vi "Initialize From File.vi"(0 "NI Build Specification_LV in":refnum<class "NI Build Specification_LV.lvclass">) -> (4 "NI Build Specification_LV out":refnum<class "NI Build Specification_LV.lvclass">)   [LabVIEW 2017, in "CL_G3_VIComponentBuilder.lvlib" / "NI Build Specification_LV.lvclass"]
doc: "Initializes the class from the configuration file.\n <MustCallParent>Parent information must be read from file therefore overrides of this method must call the parent.</MustCallParent>"
uses:
  NI Build Specification_LV.lvclass
  C:/builds/Component BuilderBT/SrcDist/Exports/Exports/Export.lvclass
  Exports/Export.lvclass/Export.ctl
  NI Build Specification_LV.lvclass/NI Build Specification_LV.ctl
  Exports/Accessors/Read Export Operation Errors.vi
  Accessors/Read Export's Build Spec Name.vi
  Exports/Accessors/Read Export Config File.vi
  Exports/Accessors/Read Component Root path.vi
  Accessors/Write Build Number XML Prop Name.vi
  Accessors/Write Display Name XML Prop Name.vi
  Accessors/Write Unique Name XML Prop Name.vi
  Accessors/Write Build Spec Type.vi
  Accessors/Write Export's Build Spec Name.vi
  Accessors/Write Target Name Containing Build Specs to Build.vi
  Exports/Accessors/Write Export Operation Errors.vi
  Accessors/Write LabVIEW Project SubBuild Spec Order.vi
  <vilib>/Utility/error.llb/Error Cluster From Error Code.vi
  Exports/Export.lvclass
  <vilib>/Utility/config.llb/NI_LVConfig.lvlib
  CL_G3_VIComponentBuilder.lvlib
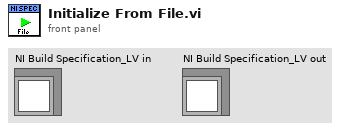
[diagram p1: front panel]
types:
  T1 = cluster{"Target Name Containing Build Specs to Build":string, "Sub Build Spec Order":path[], "Export's Build Spec Name":string}
  T2 = typedef "NI_LVConfig.lvlib/Config Data RefNum.ctl" = refnum<k1>
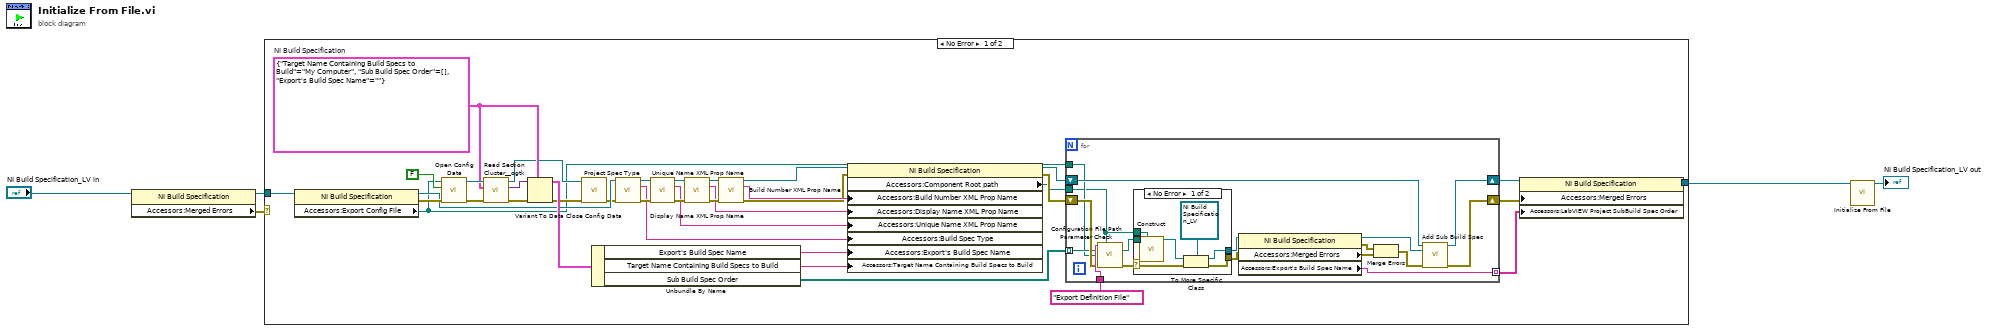
[diagram p0: block diagram]
diagram:
  n1 = property class="NI Build Specification"(reference="NI Build Specification_LV in") -> (reference out=w2:refnum<class "NI Build Specification_LV.lvclass">, "Accessors:Merged Errors"=w3:errorcluster)  [unwired: 1 in, 1 out]
  n2 = case shown="No Error" w3 {
    tunnel: [w12 w68] -> w1
    tunnel: w2 -> [w42 w68]
    frame No Error {
      w38 = T1 {"Target Name Containing Build Specs to Build"="My Computer", "Sub Build Spec Order"=[], "Export's Build Spec Name"=""}  # NI Build Specification
      n3 = property class="NI Build Specification"(reference=w42) -> (reference out=w30:refnum<class "NI Build Specification_LV.lvclass">, error out=w34:errorcluster, "Accessors:Export Config File"=w9:path)  [unwired: 1 in]
      n4 = call <vilib>:"Open Config Data.vi"("error in (no error)"=w34, "create file if necessary (T)"=FALSE, "configuration file path"=w9) -> ("error out"=w36:errorcluster, "refnum"=w40:T2)  [unwired: 6 in, 1 out]
      n5 = call <userlib>:"Read Section Cluster__ogtk.vi"("error in (no error)"=w36, "Section Formatted Cluster Type"=w38, "refnum"=w40) -> ("error out"=w35:errorcluster, "Section Formatted Cluster"=w39:variant, "dup refnum"=w33:T2)  [unwired: 4 in, 2 out]
      n6 = Variant To Data(error in=w35, type=w38, Variant=w39) -> (data=w37:T1, error out=w32:errorcluster)
      n7 = call <vilib>:"Close Config Data.vi"("error in (no error)"=w32, "refnum"=w33) -> ("error out"=w29:errorcluster)  [unwired: 8 in, 1 out]
      n8 = Unbundle By Name(w37) -> ("Export's Build Spec Name"=w8:string, "Target Name Containing Build Specs to Build"=w31:string, "Sub Build Spec Order"=w10:path[])
      n9 = call-dynamic "Project Spec Type.vi"("NI Build Specification in"=w30, "error in (no error)"=w29) -> ("NI Build Specification out"=w24:refnum<class "NI Build Specification_LV.lvclass">, "Project Specfication Type"=w17:string, "error out"=w21:errorcluster)  [unwired: 11 in]
      n10 = call-dynamic "Unique Name XML Prop Name.vi"("NI Build Specification in"=w24, "error in (no error)"=w21) -> ("NI Build Specification out"=w28:refnum<class "NI Build Specification_LV.lvclass">, "Unique Name XML Property Name"=w18:string, "error out"=w27:errorcluster)  [unwired: 11 in]
      n11 = call-dynamic "Display Name XML Prop Name.vi"("NI Build Specification in"=w28, "error in (no error)"=w27) -> ("NI Build Specification out"=w26:refnum<class "NI Build Specification_LV.lvclass">, "Display Name XML Property Name"=w19:string, "error out"=w25:errorcluster)  [unwired: 11 in]
      n12 = call-dynamic "Build Number XML Prop Name.vi"("NI Build Specification in"=w26, "error in (no error)"=w25) -> ("NI Build Specification out"=w23:refnum<class "NI Build Specification_LV.lvclass">, "Build Number XML Property Name"=w22:string, "error out"=w20:errorcluster)  [unwired: 11 in]
      n13 = property class="NI Build Specification"(reference=w23, error in=w20, "Accessors:Build Number XML Prop Name"=w22, "Accessors:Display Name XML Prop Name"=w19, "Accessors:Unique Name XML Prop Name"=w18, "Accessors:Build Spec Type"=w17, "Accessors:Export's Build Spec Name"=w8, "Accessors:Target Name Containing Build Specs to Build"=w31) -> (reference out=w15:refnum<class "NI Build Specification_LV.lvclass">, error out=w14:errorcluster, "Accessors:Component Root path"=w6:path)
      n14 = for {
        tunnel: "Export Definition File" ("Parameter Name") -> [w59]
        shift-right: [w56] -> w13
        shift-left: w15 -> [w57]
        shift-right: [w54] -> w11
        shift-left: w14 -> [w53]
        tunnel: w10 -> [w51] mode=indexing
        tunnel: w9 -> [w50]
        tunnel: [w46] -> w7 mode=indexing
        tunnel: w6 -> [w45]
        n15 = call "Configuration File Path Parameter Check.vi"("Parameter Name"=w59, "Component Root Path"=w45, "Specified Path in Configuration File"=w51, "Configuration File Path"=w50, "error in (no error)"=w53) -> ("dup Specified Path in Configuration File"=w58:path, "error out"=w52:errorcluster)  [unwired: 8 in, 1 out]
        n16 = case shown="No Error" w52 {
          selector: w52 -> [w62 w67]
          tunnel: w58 -> [w66 _]
          tunnel: [w63 _] -> w55
          tunnel: [w61 w67] -> w48
          tunnel: w45 -> [w60 _]
          frame No Error {
            n17 = call "Construct.vi"("Export Config File"=w66, "Component Root Path"=w60) -> ("Export Out"=w65:refnum<class "Export.lvclass">)  [unwired: 13 in]
            n18 = To More Specific Class(target class=refnum<class "NI Build Specification_LV.lvclass"> refnum ("reference out"), reference=w65, error in=w62) -> (specific class reference=w63:refnum<class "NI Build Specification_LV.lvclass">, error out=w61:errorcluster)
          }
          frame Error {
          }
        }
        n19 = property class="NI Build Specification"(reference=w55, error in=w48) -> (reference out=w49:refnum<class "NI Build Specification_LV.lvclass">, error out=w47:errorcluster, "Accessors:Merged Errors"=w43:errorcluster, "Accessors:Export's Build Spec Name"=w46:string)
        n20 = Merge Errors(w47, w43) -> (w44:errorcluster)
        n21 = call "Add Sub Build Spec.vi"("NI Build Specification in"=w57, "Sub Buiild Specification"=w49, "error in (no error)"=w44) -> ("NI Build Specification out"=w56:refnum<class "NI Build Specification_LV.lvclass">, "error out"=w54:errorcluster)  [unwired: 11 in]
      }
      n22 = property class="NI Build Specification"(reference=w13, "Accessors:Merged Errors"=w11, "Accessors:LabVIEW Project SubBuild Spec Order"=w7) -> (reference out=w12:refnum<class "NI Build Specification_LV.lvclass">)  [unwired: 1 in, 1 out]
    }
    frame Error {
    }
  }
  n23 = call-parent "Initialize From File.vi"("Export in"=w1) -> ("Export out"=→"NI Build Specification_LV out":refnum<class "NI Build Specification_LV.lvclass">)  [unwired: 14 in]
